vi "_Create (Friend).vi"(8 "error in (no error)":errorcluster, 11 "MapImp in":refnum<class "MapImp.lvclass">) -> (0 "error out":errorcluster, 3 "MapImp out":refnum<class "MapImp.lvclass">)   [LabVIEW 2013, in "LapDog.Collections.v_.Maps.lvlib" / "MapImp.lvclass"]
uses:
  MapImp.lvclass
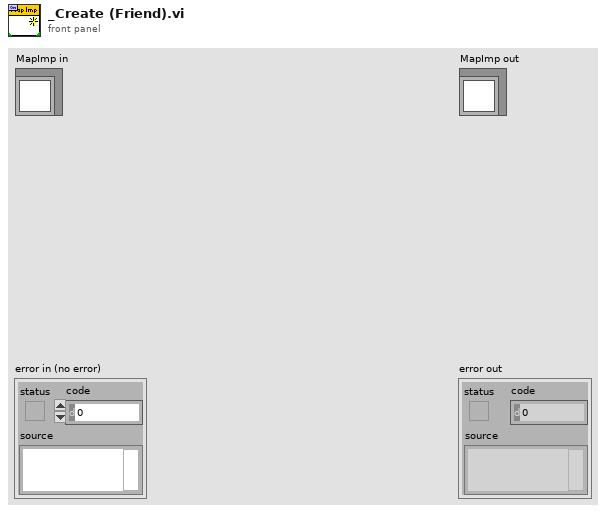
[diagram p1: front panel]
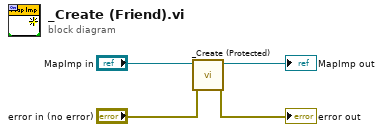
[diagram p0: block diagram]
diagram:
  n1 = call-dynamic "_Create (Protected).vi"("error in (no error)"="error in (no error)", "MapImp in"="MapImp in") -> ("error out"=→"error out":errorcluster, "MapImp out"=→"MapImp out":refnum<class "MapImp.lvclass">)  [unwired: 8 in]
